vi "Set imaging buffer.vi"(6 "Image type":u32, 8 "error in (no error)":errorcluster, 9 "Buffer 2":u16[][](array[numeric]), 10 "Buffer":T1, 11 "DAQMH121119OrcaFlash in":refnum<class "DAQOrcaFlash.lvclass">) -> (0 "error out":errorcluster, 3 "DAQMH121119OrcaFlash out":refnum<class "DAQOrcaFlash.lvclass">)   [LabVIEW 2012, in "DAQOrcaFlash.lvclass"]
uses:
  DAQOrcaFlash.lvclass
  DAQOrcaFlash.lvclass/DAQOrcaFlash.ctl
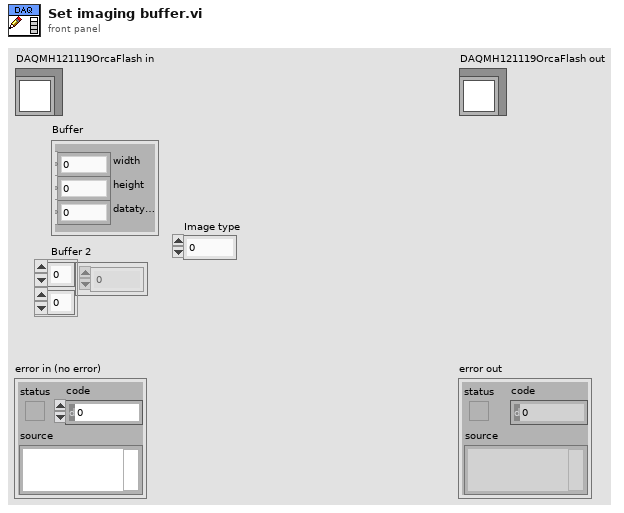
[diagram p1: front panel]
types:
  T1 = cluster{"width":u32, "height":u32, "datatype":u32}
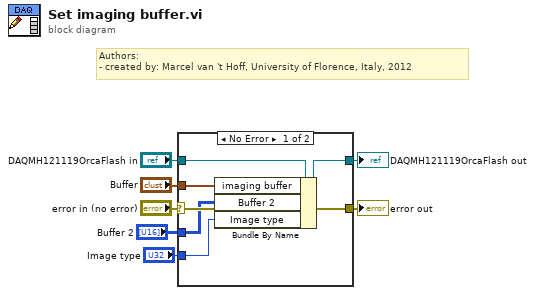
[diagram p0: block diagram]
diagram:
  # "Authors: \n- created by: Marcel van 't Hoff, University of Florence, Italy, 2012"
  n1 = case shown="No Error" "error in (no error)" {
    selector: "error in (no error)" -> [w13 w15]
    tunnel: [w13 w15] -> w6
    tunnel: [w11 w14] -> w4
    tunnel: "DAQMH121119OrcaFlash in" -> [w12 w14]
    tunnel: "Buffer" -> [w10 _]
    tunnel: "Buffer 2" -> [w9 _]
    tunnel: "Image type" -> [w8 _]
    frame No Error {
      n2 = Bundle By Name(cluster=w12, "imaging buffer"=w10, "Buffer 2"=w9, "Image type"=w8) -> (w11:refnum<class "DAQOrcaFlash.lvclass">)
    }
    frame Error {
    }
  }
  "error out" <- w6
  "DAQMH121119OrcaFlash out" <- w4
